vi "Wite_1D_Array_As_String.vi"(6 "Precision":i16, 7 "File Path":path, 8 "append to file? (new file:F)":bool=TRUE, 9 "Comparison Array":dbl[](array[numeric]), 10 "1st Column Text":string, 11 "1D Array":dbl[](array[numeric])) -> (3 "File Path Out":path)   [LabVIEW 2011]
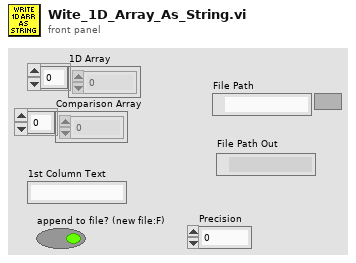
[diagram p1: front panel]
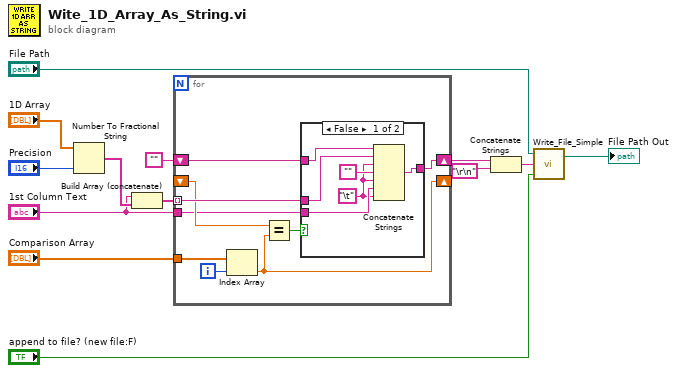
[diagram p0: block diagram]
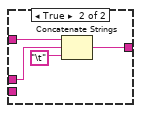
[diagram p2: hidden frame]
diagram:
  n1 = Number To Fractional String(number="1D Array", precision (6)="Precision") -> (F-format string=w6:string[])  [unwired: 2 in]
  n2 = Build Array (concatenate)("1st Column Text", w6) -> (w12:string[])
  n3 = for {
    shift-right: [w21] -> w8
    shift-left: "" -> [w22]
    tunnel: w12 -> [w20] mode=indexing
    shift-right: [w14] -> _
    shift-left: _ -> [w19]
    tunnel: "Comparison Array" -> [w16]
    tunnel: "1st Column Text" -> [w17]
    i -> [w15]
    n4 = Index Array(array=w16, index=w15) -> (element=w14:dbl)
    n5 = Equal?(x=w19, y=w14) -> (x = y?=w18:bool)
    n6 = case shown="False" w18 {
      tunnel: w22 -> [w25 w32]
      tunnel: [w28 w31] -> w21
      tunnel: w20 -> [w27 w30]
      tunnel: w17 -> [w24 _]
      frame False {
        w23 = "\t"
        n7 = Concatenate Strings(w25, w27, w23, "", w23, w24, w23) -> (w28:string)
      }
      frame True {
        n8 = Concatenate Strings(w32, w30, "\t") -> (w31:string)
      }
    }
  }
  n9 = Concatenate Strings(w8, "\r\n") -> (w7:string)
  n10 = call "Write_File_Simple.vi"("append to file? (new file:F)"="append to file? (new file:F)", "character string"=w7, "file path"="File Path") -> ("file path Out"=→"File Path Out":path)  [unwired: 1 out]
